vi "List Elements (byCategory).vi"(9 "category":string, 11 "Datastore.Dictionaries in":refnum<class "Datastore.Dictionaries.lvclass">) -> (0 "elements":string[](array[string]), 1 "category dup":string, 3 "Datastore.Dictionaries":refnum<class "Datastore.Dictionaries.lvclass">, 4 "found?":bool)   [LabVIEW 2021, in "Bananas.lvlib" / "Datastore.Dictionaries.lvclass"]
uses:
  Datastore.Dictionaries.lvclass
  Datastore.Dictionaries.lvclass/Datastore.Dictionaries.ctl
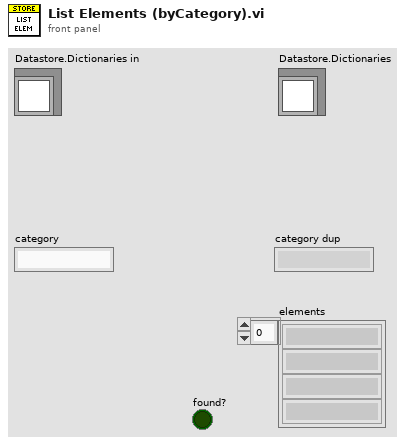
[diagram p1: front panel]
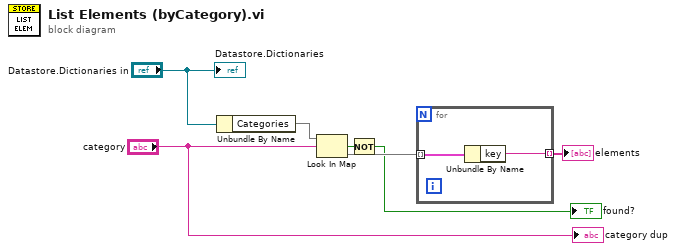
[diagram p0: block diagram]
diagram:
  n1 = Unbundle By Name("Datastore.Dictionaries in") -> ("Categories"=w6:map{string, map{string, variant}})
  n2 = Look In Map(map=w6, key="category") -> (key not found?=w2:bool, value=w5:map{string, variant})  [unwired: 1 in]
  n3 = Not(x=w2) -> (.not. x?=→"found?":bool)
  n4 = for {
    tunnel: w5 -> [w9] mode=indexing
    tunnel: [w8] -> w7 mode=indexing
    n5 = Unbundle By Name(w9) -> ("key"=w8:string)
  }
  "elements" <- w7
  "Datastore.Dictionaries" <- "Datastore.Dictionaries in"
  "category dup" <- "category"
